vi "In Subpanel.vi"(11 "VI Ref":refnum<vi>) -> (3 "VI in SubPanel?":bool)   [LabVIEW 2023]
doc: "Determine if VI is running in a subpanel. If VI ref is not wired, the calling VI's ref is used."
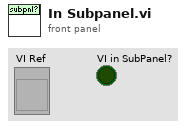
[diagram p1: front panel]
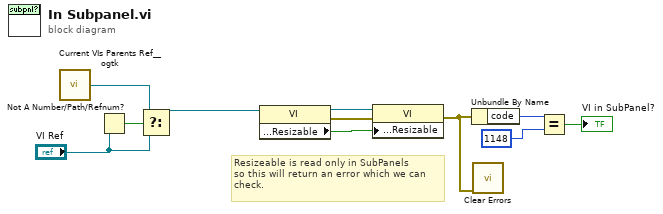
[diagram p0: block diagram]
diagram:
  # "Resizeable is read only in SubPanels\nso this will return an error which we can\ncheck."
  n1 = call <userlib>:"Current VIs Parents Ref__ogtk.vi"() -> ("Calling VI's Reference"=w4:refnum<vi>)  [unwired: 2 in]
  n2 = Not A Number/Path/Refnum?(number/path/refnum="VI Ref") -> (NaN/Path/Refnum?=w5:bool)
  n3 = Select(t=w4, s=w5, f="VI Ref") -> (s? t:f=w3:refnum<vi>)
  n4 = property class="VI"(reference=w3) -> (reference out=w10:refnum<vi>, error out=w11:errorcluster, "Front Panel Window:Resizable"=w9:bool)  [unwired: 1 in]
  n5 = property class="VI"(reference=w10, error in=w11, "Front Panel Window:Resizable"=w9) -> (error out=w1:errorcluster)  [unwired: 1 out]
  n6 = Unbundle By Name(w1) -> ("code"=w6:i32)
  n7 = call <vilib>:"Clear Errors.vi"("error in (no error)"=w1) -> ()  [unwired: 5 in, 2 out]
  n8 = Equal?(x=w6, y=1148) -> (x = y?=→"VI in SubPanel?":bool)
